vi "Select Between Expanded Pin Information Options.vi"(0 "Current":T1, 1 "Pins and/or Pin Groups Information":T3[](array[typedef]), 5 "Duplicate":T1) -> (4 "Best Choice Out":T1)   [LabVIEW 2019]
uses:
  TSM Expanded Pin Information.ctl
  TSM Pin Type Identifier.ctl
  TSM Pin Information.ctl
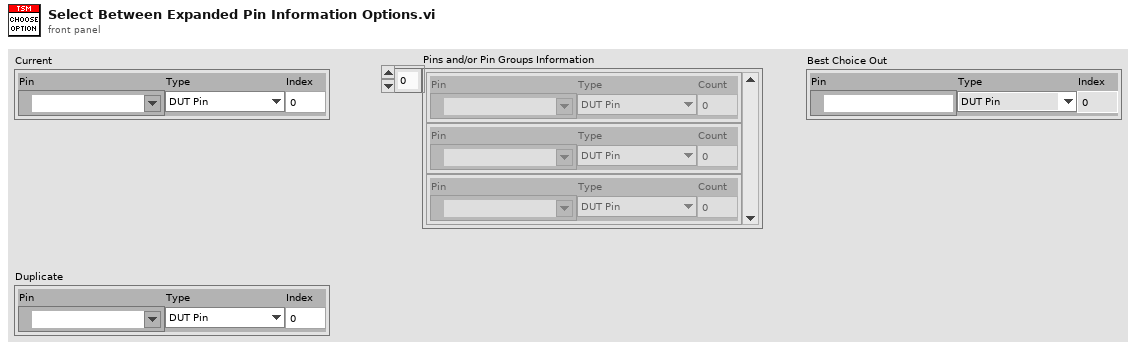
[diagram p1: front panel]
types:
  T1 = typedef "TSM Expanded Pin Information.ctl" = cluster{"Pin":tag, "Type":T2, "Index":i32}
  T2 = typedef "TSM Pin Type Identifier.ctl" = enum8{"DUT Pin", "System Pin", "Pin Group", "Not Determined"}
  T3 = typedef "TSM Pin Information.ctl" = cluster{"Pin":tag, "Type":T2, "Count":i32}
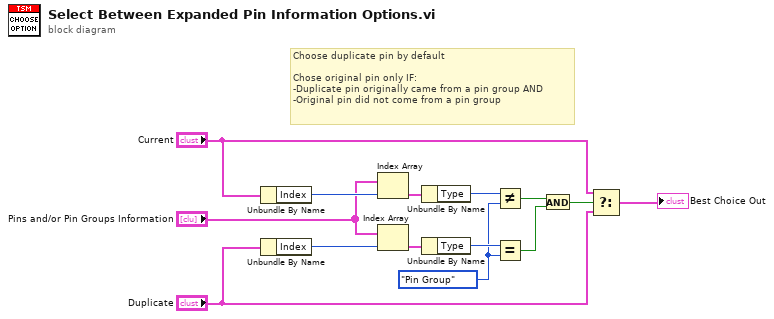
[diagram p0: block diagram]
diagram:
  w1 = TSM_Pin_Type_Identifier."Pin Group" ("y")
  # "Choose duplicate pin by default\n\nChose original pin only IF:\n-Duplicate pin originally came from a pin group AND\n-Original pin did not come from a pin group"
  n1 = Unbundle By Name("Current") -> ("Index"=w14:i32)
  n2 = Unbundle By Name("Duplicate") -> ("Index"=w13:i32)
  n3 = Index Array(array="Pins and/or Pin Groups Information", index=w14) -> (element=w11:T3)
  n4 = Index Array(array="Pins and/or Pin Groups Information", index=w13) -> (element=w10:T3)
  n5 = Unbundle By Name(w11) -> ("Type"=w6:T2)
  n6 = Unbundle By Name(w10) -> ("Type"=w5:T2)
  n7 = Not Equal?(x=w6, y=w1) -> (x != y?=w4:bool)
  n8 = Equal?(x=w5, y=w1) -> (x = y?=w3:bool)
  n9 = And(x=w4, y=w3) -> (x .and. y?=w2:bool)
  n10 = Select(t="Current", s=w2, f="Duplicate") -> (s? t:f=→"Best Choice Out":T1)
